vi "sm.main-sm.vi"() -> ()   [LabVIEW 2019]
uses:
  <vilib>/rvi/Emulation/niFpgaSctlEmulationGetInTimedLoop.vi
  <vilib>/rvi/Emulation/niFpgaEmulationIsFPGAContextNoSignature.vi
  <vilib>/rvi/DataTransferAndStorage/Container/Common/niFpgaContainerGetUniqueNameForEmu.vi
  <vilib>/rvi/Memory/Memory_Emulation/niFpgaMemoryEmulationCacheClearOnFirstRun.vi
  <vilib>/rvi/Memory/Memory_Emulation/nirvimemoryEmulationManagerCache_MakeExclusive.vi
  <vilib>/rvi/Memory/Memory_Emulation/niFpgaMemoryEmulationValidateCache.vi
  <vilib>/rvi/Memory/Memory_Emulation/nirvimemoryEmulationManagerCache_InsertValue.vi
  <vilib>/Utility/error.llb/Clear Errors.vi
  <vilib>/rvi/Memory/Memory_Emulation/nirvimemoryEmulationManagerCache_ReleaseExclusive.vi
  <vilib>/rvi/Memory/Memory_Emulation/nirvimemoryEmulationManagerCache_GetValue.vi
  <vilib>/rvi/Memory/Memory_Emulation/nirvimemoryEmulationManagerCache_SetValue.vi
  <vilib>/rvi/Emulation/niFpgaProcessEmulError.vi
  rti.global.vi
  <vilib>/rvi/DataTransferAndStorage/Container/XNode/niFpgaContainer.xnode
  <vilib>/rvi/DataTransferAndStorage/Register/Emulation/niFpgaRegisterEmulation.vi
panel:
  out "home sensor":bool
  out "sub-mode":u8
  out "mode":u8
  out "mode req":u8
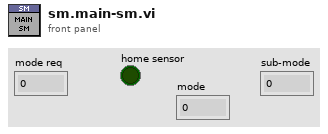
[diagram p1: front panel]
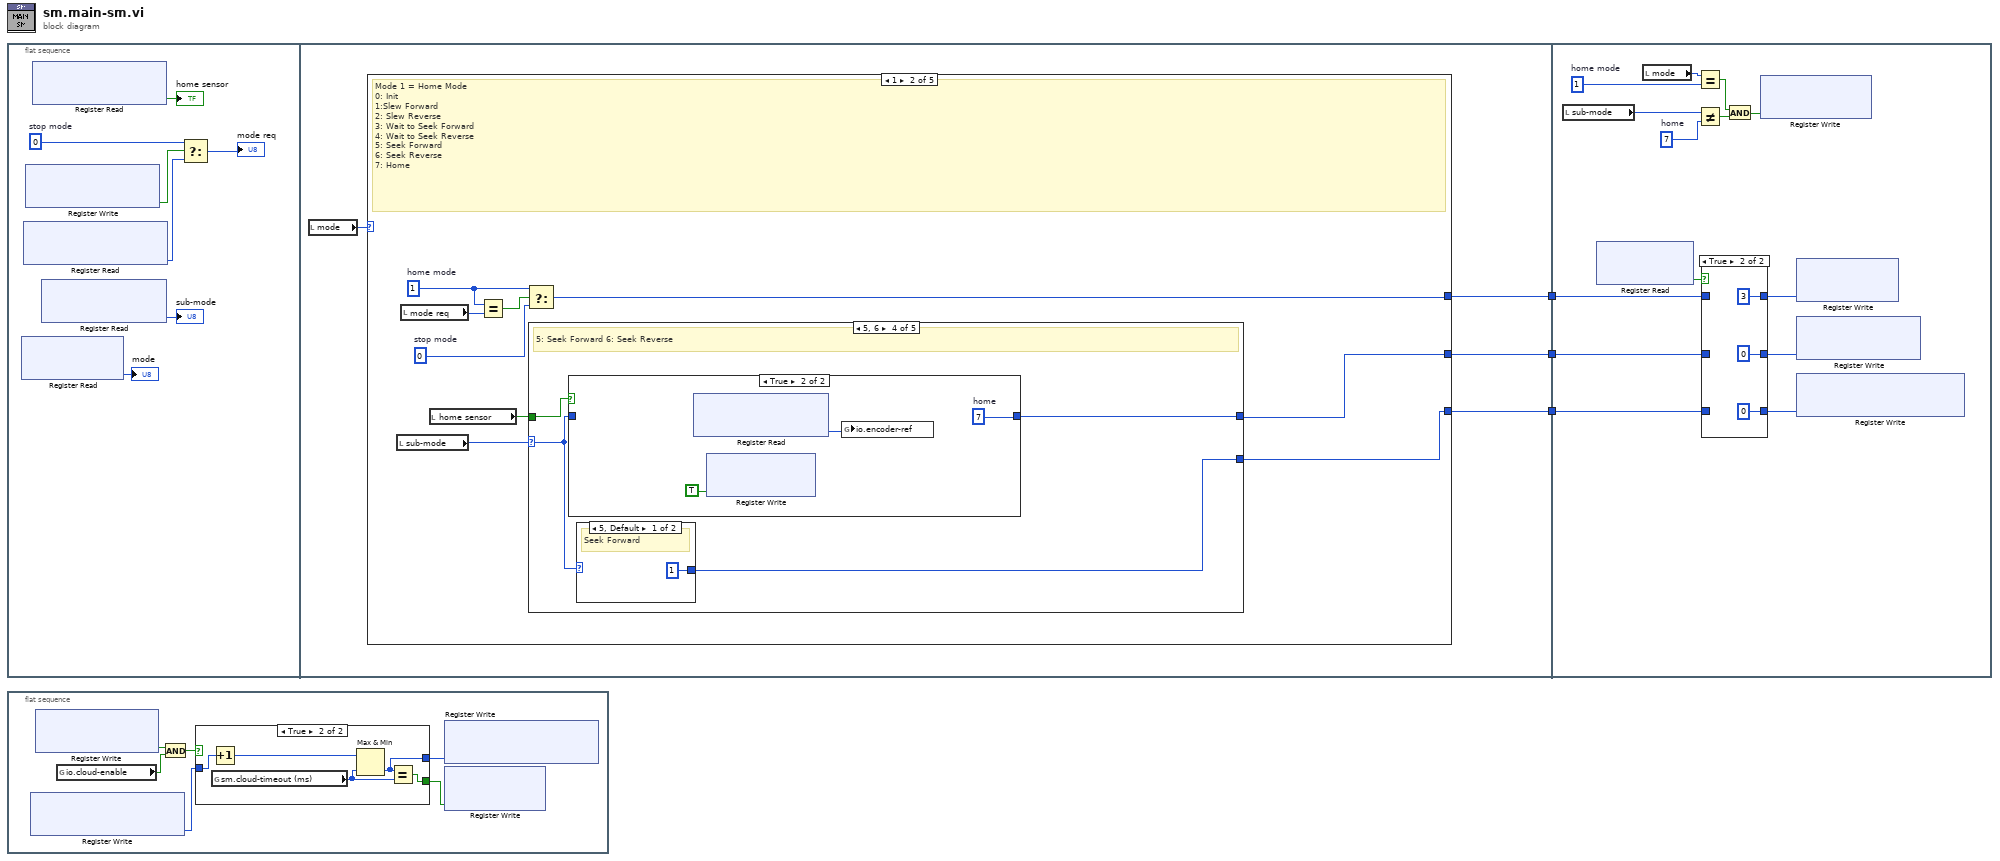
[diagram p0: block diagram]
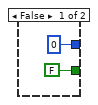
[diagram p2: hidden frame]
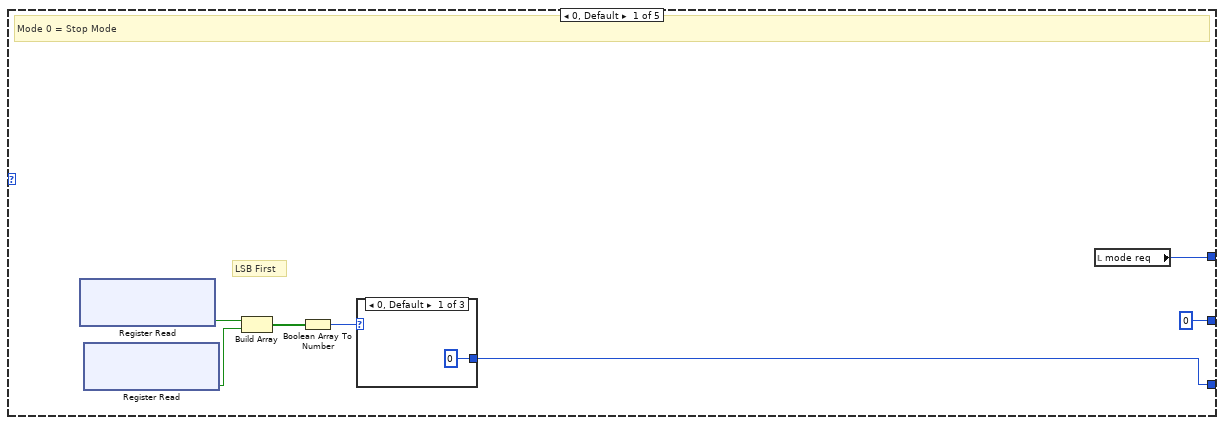
[diagram p3: hidden frame]
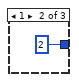
[diagram p4: hidden frame]
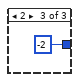
[diagram p5: hidden frame]
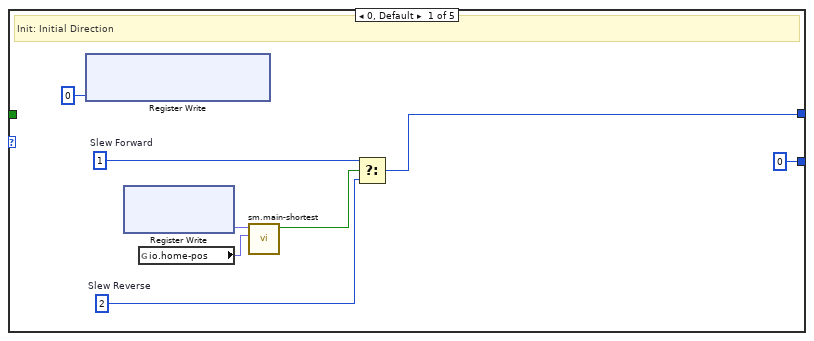
[diagram p6: hidden frame]
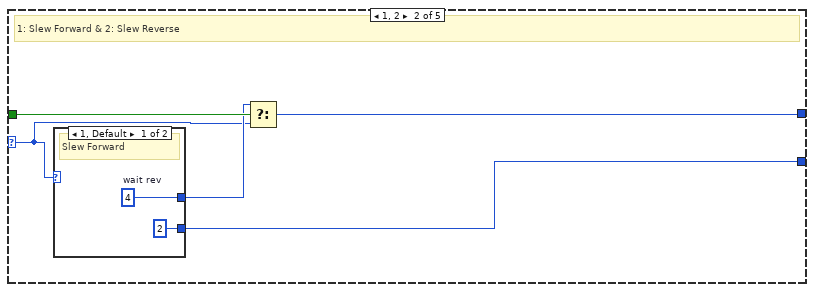
[diagram p7: hidden frame]
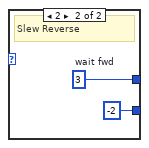
[diagram p8: hidden frame]
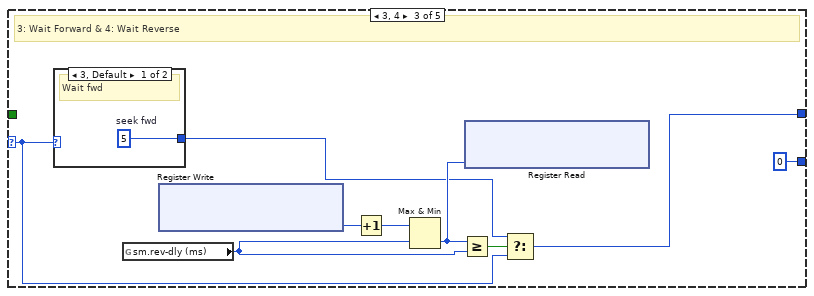
[diagram p9: hidden frame]
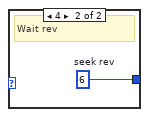
[diagram p10: hidden frame]
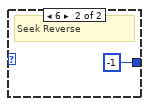
[diagram p12: hidden frame]
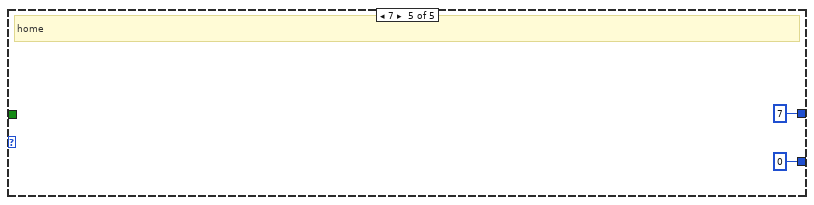
[diagram p13: hidden frame]
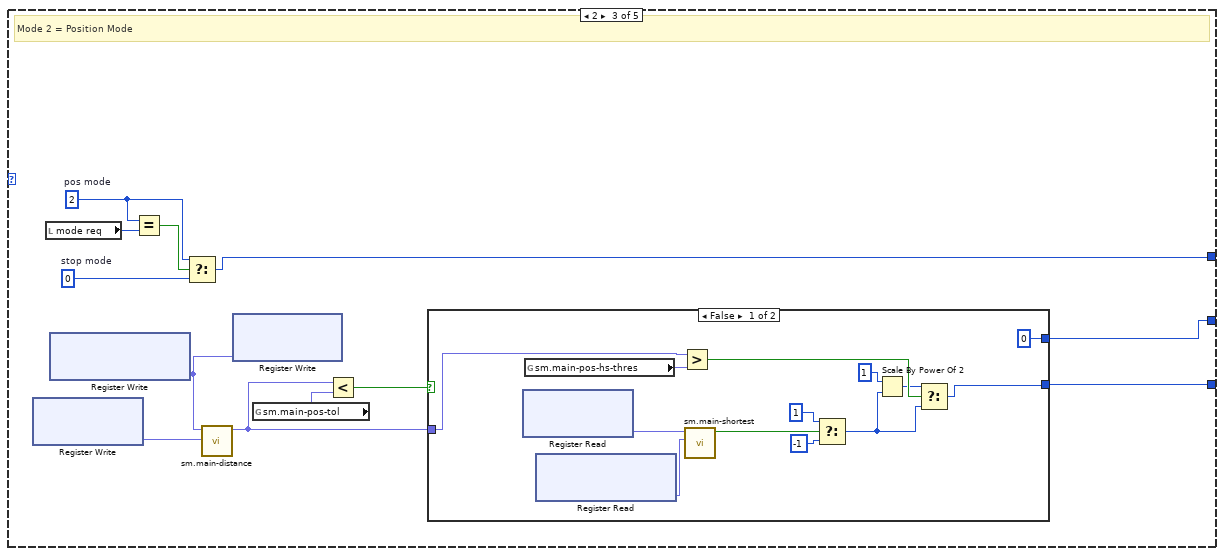
[diagram p14: hidden frame]
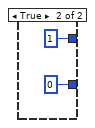
[diagram p15: hidden frame]
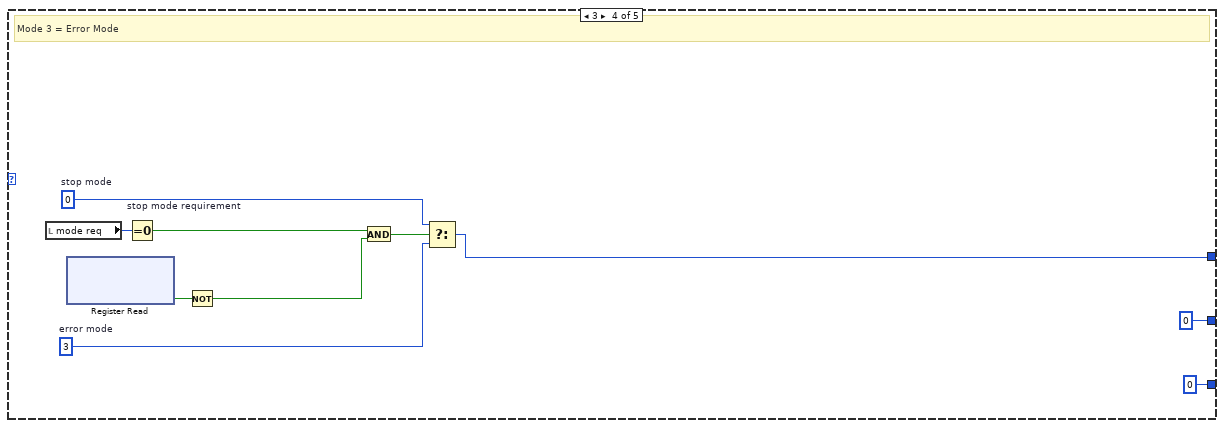
[diagram p16: hidden frame]
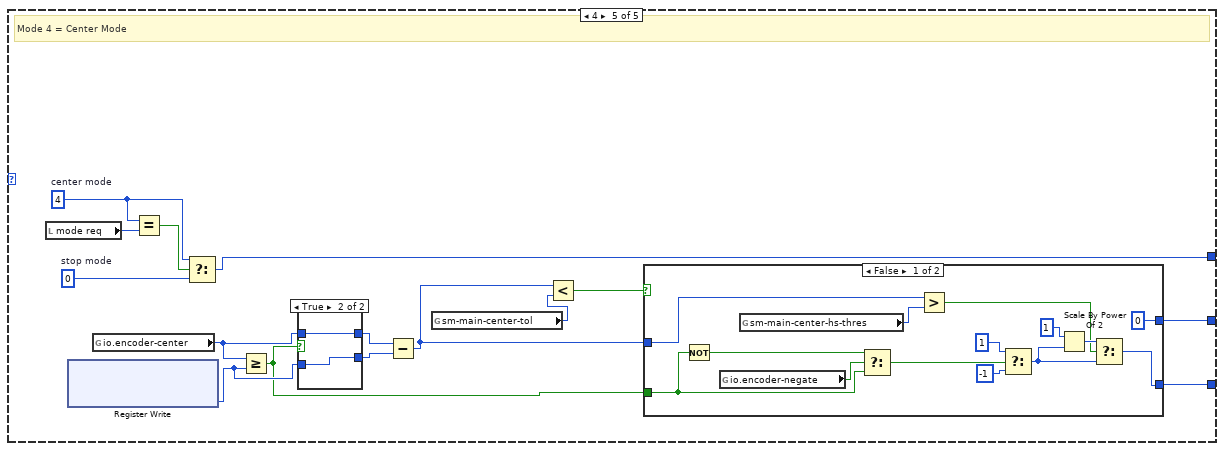
[diagram p17: hidden frame]
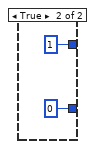
[diagram p18: hidden frame]
diagram:
  n1 = flat-sequence {
    tunnel: [w14] -> w3
    tunnel: [w13] -> w2
    tunnel: [w12] -> w1
    tunnel: w3 -> [w155]
    tunnel: w2 -> [w157]
    tunnel: w1 -> [w153]
    frame #0 {
      w5 = u8 0  # stop mode
      n2 = xnode "Register Read"() -> ("Data"=→"mode":u8)  [unwired: 1 in, 1 out]
      n3 = xnode "Register Read"() -> ("Data"=w6:u8)  [unwired: 1 in, 1 out]
      n4 = xnode "Register Write"() -> ("Data"=w7:bool)  [unwired: 1 in, 1 out]
      n5 = xnode "Register Read"() -> ("Data"=→"home sensor":bool)  [unwired: 1 in, 1 out]
      n6 = xnode "Register Read"() -> ("Data"=→"sub-mode":u8)  [unwired: 1 in, 1 out]
      n7 = Select(t=w5, s=w7, f=w6) -> (s? t:f=→"mode req":u8)
    }
    frame #1 {
      n8 = local read "mode"() -> (w11:u8)
      n9 = case shown="1" w11 {
        tunnel: [w17 w28 w81 i8 0 ("Data") w118] -> w13
        tunnel: [w16 w31 w83 w106 w113] -> w14
        tunnel: [u8 0 ("Data") w29 w79 u8 0 ("Data") w119] -> w12
        frame 0, Default {
          # "LSB First"
          # "Mode 0 = Stop Mode"
          n10 = xnode "Register Read"() -> ("Data"=w20:bool)  [unwired: 1 in, 1 out]
          n11 = xnode "Register Read"() -> ("Data"=w19:bool)  [unwired: 1 in, 1 out]
          n12 = Build Array(w20, w19) -> (w21:bool[])
          n13 = Boolean Array To Number(Boolean array=w21) -> (number=w18:u8)
          n14 = case shown="0, Default" w18 {
            tunnel: [i8 0 ("Data") i8 2 ("Data") i8 -2 ("Data")] -> w17
            frame 0, Default {
            }
            frame 1 {
            }
            frame 2 {
            }
          }
          n15 = local read "mode req"() -> (w16:u8)
        }
        frame 1 {
          w32 = u8 0  # stop mode
          w25 = u8 1  # home mode
          # "Mode 1 = Home Mode\n0: Init\n1:Slew Forward\n2: Slew Reverse\n3: Wait to Seek Forward\n4: Wait to Seek Reverse\n5: Seek Forward\n6: Seek Reverse\n7: Home"
          n16 = local read "sub-mode"() -> (w30:u8)
          n17 = local read "mode req"() -> (w26:u8)
          n18 = local read "home sensor"() -> (w27:bool)
          n19 = Equal?(x=w25, y=w26) -> (x = y?=w33:bool)
          n20 = Select(t=w25, s=w33, f=w32) -> (s? t:f=w31:u8)
          n21 = case shown="5, 6" w30 {
            selector: w30 -> [_ w42 w54 w62 _]
            tunnel: [w35 w45 w52 w64 u8 7 ("Data")] -> w29
            tunnel: w27 -> [_ w46 _ w63 _]
            tunnel: [i8 0 ("Data") w43 i8 0 ("Data") w65 i8 0 ("Data")] -> w28
            frame 0, Default {
              w36 = u8 2  # Slew Reverse
              w37 = u8 1  # Slew Forward
              # "Init: Initial Direction"
              n22 = xnode "Register Write"("Data"=u32 0) -> ()  [unwired: 1 in, 1 out]
              n23 = xnode "Register Write"() -> ("Data"=w40:fxp<+/-,32,2>)  [unwired: 1 in, 1 out]
              n24 = global read "rti.global.vi" "io.home-pos"() -> (w39:fxp<+/-,32,2>)
              n25 = call "sm.main-shortest.vi"("destination"=w39, "origin"=w40) -> ("forward?"=w38:bool)  [unwired: 9 in]
              n26 = Select(t=w37, s=w38, f=w36) -> (s? t:f=w35:u8)
            }
            frame 1, 2 {
              # "1: Slew Forward & 2: Slew Reverse"
              n27 = case shown="1, Default" w42 {
                tunnel: [w48 w50] -> w44
                tunnel: [i8 2 ("Data") i8 -2 ("Data")] -> w43
                frame 1, Default {
                  w48 = u8 4  # wait rev
                  # "Slew Forward"
                }
                frame 2 {
                  w50 = u8 3  # wait fwd
                  # "Slew Reverse"
                }
              }
              n28 = Select(t=w44, s=w46, f=w42) -> (s? t:f=w45:u8)
            }
            frame 3, 4 {
              # "3: Wait Forward & 4: Wait Reverse"
              n29 = case shown="3, Default" w54 {
                tunnel: [w60 w61] -> w53
                frame 3, Default {
                  w60 = u8 5  # seek fwd
                  # "Wait fwd"
                }
                frame 4 {
                  w61 = u8 6  # seek rev
                  # "Wait rev"
                }
              }
              n30 = global read "rti.global.vi" "sm.rev-dly (ms)"() -> (w57:u32)
              n31 = xnode "Register Write"() -> ("Data"=w58:u32)  [unwired: 1 in, 1 out]
              n32 = Increment(x=w58) -> (x+1=w59:u32)
              n33 = Max & Min(x=w59, y=w57) -> (min(x,y)=w56:u32)  [unwired: 1 out]
              n34 = Greater Or Equal?(x=w56, y=w57) -> (x >= y?=w55:bool)
              n35 = xnode "Register Read"("Data"=w56) -> ()  [unwired: 1 in, 1 out]
              n36 = Select(t=w53, s=w55, f=w54) -> (s? t:f=w52:u8)
            }
            frame 5, 6 {
              # "5: Seek Forward 6: Seek Reverse"
              n37 = case shown="True" w63 {
                tunnel: [w66 w68] -> w64
                tunnel: w62 -> [w66 _]
                frame False {
                }
                frame True {
                  w68 = u8 7  # home
                  n38 = xnode "Register Read"() -> ("Data"=w69:u64)  [unwired: 1 in, 1 out]
                  n39 = xnode "Register Write"("Data"=TRUE) -> ()  [unwired: 1 in, 1 out]
                  n40 = global write "rti.global.vi" "io.encoder-ref"(w69) -> ()
                }
              }
              n41 = case shown="5, Default" w62 {
                tunnel: [i8 1 ("Data") i8 -1 ("Data")] -> w65
                frame 5, Default {
                  # "Seek Forward"
                }
                frame 6 {
                  # "Seek Reverse"
                }
              }
            }
            frame 7 {
              # "home"
            }
          }
        }
        frame 2 {
          w84 = u8 0  # stop mode
          w74 = u8 2  # pos mode
          # "Mode 2 = Position Mode"
          n42 = xnode "Register Write"() -> ("Data"=w82:fxp<+/-,32,2>)  [unwired: 1 in, 1 out]
          n43 = local read "mode req"() -> (w75:u8)
          n44 = xnode "Register Write"() -> ("Data"=w77:fxp<+/-,32,2>)  [unwired: 1 in, 1 out]
          n45 = Equal?(x=w74, y=w75) -> (x = y?=w85:bool)
          n46 = Select(t=w74, s=w85, f=w84) -> (s? t:f=w83:u8)
          n47 = call "sm.main-distance.vi"("y"=w82, "x"=w77) -> ("distance"=w80:fxp<+/-,32,2>)  [unwired: 9 in]
          n48 = xnode "Register Write"("Data"=w77) -> ()  [unwired: 1 in, 1 out]
          n49 = global read "rti.global.vi" "sm.main-pos-tol"() -> (w78:fxp<+/-,32,2>)
          n50 = Less?(x=w80, y=w78) -> (x < y?=w76:bool)
          n51 = case shown="False" w76 {
            tunnel: [w88 i8 0 ("Data")] -> w81
            tunnel: w80 -> [w93 _]
            tunnel: [u8 0 ("Data") u8 1 ("Data")] -> w79
            frame False {
              n52 = xnode "Register Read"() -> ("Data"=w97:fxp<+/-,32,2>)  [unwired: 1 in, 1 out]
              n53 = global read "rti.global.vi" "sm.main-pos-hs-thres"() -> (w86:fxp<+/-,32,2>)
              n54 = xnode "Register Read"() -> ("Data"=w98:fxp<+/-,32,2>)  [unwired: 1 in, 1 out]
              n55 = Greater?(x=w93, y=w86) -> (0:w92:bool)
              n56 = call "sm.main-shortest.vi"("destination"=w98, "origin"=w97) -> ("forward?"=w96:bool)  [unwired: 9 in]
              n57 = Select(t=i8 1 ("Data"), s=w96, f=i8 -1) -> (s? t:f=w90:i8)
              n58 = Scale By Power Of 2(n=i16 1, x=w90) -> (x*2^n=w89:i8)
              n59 = Select(t=w89, s=w92, f=w90) -> (s? t:f=w88:i8)
            }
            frame True {
            }
          }
        }
        frame 3 {
          w107 = u8 3  # error mode
          w108 = u8 0  # stop mode
          # "Mode 3 = Error Mode"
          n60 = local read "mode req"() -> (w109:u8)
          n61 = xnode "Register Read"() -> ("Data"=w104:bool)  [unwired: 1 in, 1 out]
          n62 = Equal To 0? "stop mode requirement"(x=w109) -> (x = 0?=w103:bool)
          n63 = Not(x=w104) -> (.not. x?=w102:bool)
          n64 = And(x=w103, y=w102) -> (x .and. y?=w101:bool)
          n65 = Select(t=w108, s=w101, f=w107) -> (s? t:f=w106:u8)
        }
        frame 4 {
          w114 = u8 0  # stop mode
          w111 = u8 4  # center mode
          # "Mode 4 = Center Mode"
          n66 = local read "mode req"() -> (w112:u8)
          n67 = xnode "Register Write"() -> ("Data"=w124:u64)  [unwired: 1 in, 1 out]
          n68 = global read "rti.global.vi" "io.encoder-center"() -> (w125:u64)
          n69 = Equal?(x=w111, y=w112) -> (x = y?=w115:bool)
          n70 = Select(t=w111, s=w115, f=w114) -> (s? t:f=w113:u8)
          n71 = Greater Or Equal?(x=w125, y=w124) -> (x >= y?=w116:bool)
          n72 = case shown="True" w116 {
            tunnel: w125 -> [w143 w145]
            tunnel: w124 -> [w142 w144]
            tunnel: [w142 w145] -> w123
            tunnel: [w143 w144] -> w122
            frame False {
            }
            frame True {
            }
          }
          n73 = Subtract(x=w123, y=w122) -> (x-y=w117:u64)
          n74 = global read "rti.global.vi" "sm-main-center-tol"() -> (w121:u64)
          n75 = Less?(x=w117, y=w121) -> (x < y?=w120:bool)
          n76 = case shown="False" w120 {
            tunnel: [u8 0 ("Data") u8 1 ("Data")] -> w119
            tunnel: [w130 i8 0 ("f")] -> w118
            tunnel: w117 -> [w137 _]
            tunnel: w116 -> [w128 _]
            frame False {
              n77 = Not(x=w128) -> (.not. x?=w127:bool)
              n78 = global read "rti.global.vi" "io.encoder-negate"() -> (w129:bool)
              n79 = global read "rti.global.vi" "sm-main-center-hs-thres"() -> (w138:u64)
              n80 = Select(t=w127, s=w129, f=w128) -> (s? t:f=w126:bool)
              n81 = Greater?(x=w137, y=w138) -> (0:w131:bool)
              n82 = Select(t=i8 1 ("Data"), s=w126, f=i8 -1) -> (s? t:f=w133:i8)
              n83 = Scale By Power Of 2(n=i16 1, x=w133) -> (x*2^n=w132:i8)
              n84 = Select(t=w132, s=w131, f=w133) -> (s? t:f=w130:i8)
            }
            frame True {
            }
          }
        }
      }
    }
    frame #2 {
      w148 = u8 7  # home
      w151 = u8 1  # home mode
      n85 = local read "sub-mode"() -> (w149:u8)
      n86 = xnode "Register Read"() -> ("Data"=w159:bool)  [unwired: 1 in, 1 out]
      n87 = local read "mode"() -> (w152:u8)
      n88 = Equal?(x=w152, y=w151) -> (x = y?=w150:bool)
      n89 = Not Equal?(x=w149, y=w148) -> (x != y?=w147:bool)
      n90 = case shown="True" w159 {
        tunnel: [w162 i8 0 ("Data")] -> w158
        tunnel: w157 -> [w162 _]
        tunnel: [w161 u8 3 ("f")] -> w156
        tunnel: w155 -> [w161 _]
        tunnel: [w160 u8 0 ("Data")] -> w154
        tunnel: w153 -> [w160 _]
        frame False {
        }
        frame True {
        }
      }
      n91 = And(x=w150, y=w147) -> (x .and. y?=w146:bool)
      n92 = xnode "Register Write"("Data"=w146) -> ()  [unwired: 1 in, 1 out]
      n93 = xnode "Register Write"("Data"=w156) -> ()  [unwired: 1 in, 1 out]
      n94 = xnode "Register Write"("Data"=w154) -> ()  [unwired: 1 in, 1 out]
      n95 = xnode "Register Write"("Data"=w158) -> ()  [unwired: 1 in, 1 out]
    }
  }
  n96 = flat-sequence {
    frame #0 {
      n97 = xnode "Register Write"() -> ("Data"=w169:u32)  [unwired: 1 in, 1 out]
      n98 = xnode "Register Write"() -> ("Data"=w168:bool)  [unwired: 1 in, 1 out]
      n99 = global read "rti.global.vi" "io.cloud-enable"() -> (w166:bool)
      n100 = And(x=w168, y=w166) -> (x .and. y?=w167:bool)
      n101 = case shown="True" w167 {
        tunnel: w169 -> [_ w178]
        tunnel: [u32 0 ("Data") w175] -> w170
        tunnel: [FALSE w174] -> w171
        frame False {
        }
        frame True {
          n102 = Increment(x=w178) -> (x+1=w177:u32)
          n103 = global read "rti.global.vi" "sm.cloud-timeout (ms)"() -> (w176:u32)
          n104 = Max & Min(x=w177, y=w176) -> (min(x,y)=w175:u32)  [unwired: 1 out]
          n105 = Equal?(x=w175, y=w176) -> (x = y?=w174:bool)
        }
      }
      n106 = xnode "Register Write"("Data"=w170) -> ()  [unwired: 1 in, 1 out]
      n107 = xnode "Register Write"("Data"=w171) -> ()  [unwired: 1 in, 1 out]
    }
  }
